vi "AutoIntakeRear.vi"() -> ()   [LabVIEW 2015]
uses:
  Typedef/IntakeControllerActions.ctl
  Typedef/IntakeControllerMsg.ctl
  ArmController/ArmController.lvlib
panel:
  in  "milliseconds to wait 2":u32=500
  in  "milliseconds to wait":u32=600
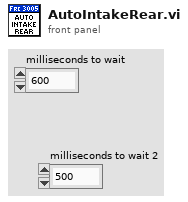
[diagram p1: front panel]
types:
  T1 = typedef "IntakeControllerMsg.ctl" = cluster{"Cmd":T2, "Data":variant}
  T2 = typedef "IntakeControllerActions.ctl" = enum16{"Wait on Intake Rear", "Wait on Angle Rear", "Go To Angle Rear", "Wait on Intake Front", "Wait on Angle Front", "Set Roller Front", "Set Roller Rear", "Go To Angle Front", "Wait ms"}
  T3 = cluster{"Down":dbl, "Pickup":dbl, "Shoot":dbl, "Turtle":dbl, "Intake Block":dbl, "Intake Transfer":dbl}
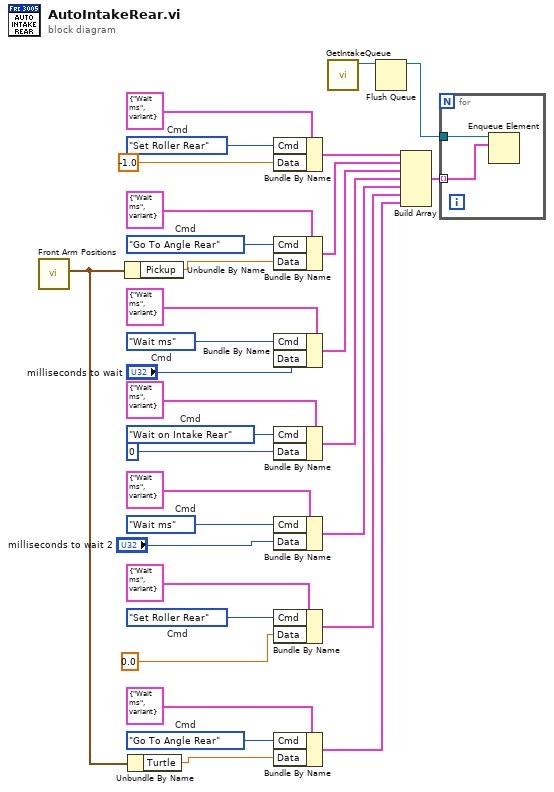
[diagram p0: block diagram]
diagram:
  w32 = IntakeControllerActions."Go To Angle Rear"  # Cmd
  w23 = IntakeControllerActions."Set Roller Rear"  # Cmd
  w27 = IntakeControllerActions."Wait ms"  # Cmd
  w20 = IntakeControllerActions."Wait on Intake Rear"  # Cmd
  w14 = IntakeControllerActions."Wait ms"  # Cmd
  w11 = IntakeControllerActions."Go To Angle Rear"  # Cmd
  w8 = IntakeControllerActions."Set Roller Rear"  # Cmd
  n1 = call "Front Arm Positions.vi"() -> ("Rear Arm"=w1:T3)  [unwired: 10 in, 1 out]
  n2 = Unbundle By Name(w1) -> ("Pickup"=w3:dbl)
  n3 = Unbundle By Name(w1) -> ("Turtle"=w2:dbl)
  n4 = Bundle By Name(cluster=T1 {"Cmd"=enum."Wait ms", "Data"=variant(i32 50)} ("output cluster"), "Cmd"=w8, "Data"=-1.0 ("Diffs")) -> (w10:T1)
  n5 = Bundle By Name(cluster=T1 {"Cmd"=enum."Wait ms", "Data"=variant(i32 50)} ("output cluster"), "Cmd"=w11, "Data"=w3) -> (w13:T1)
  n6 = Bundle By Name(cluster=T1 {"Cmd"=enum."Wait ms", "Data"=variant(i32 50)} ("output cluster"), "Cmd"=w14, "Data"="milliseconds to wait") -> (w17:T1)
  n7 = Bundle By Name(cluster=T1 {"Cmd"=enum."Wait ms", "Data"=variant(i32 50)} ("output cluster"), "Cmd"=w20, "Data"=u32 0 ("milliseconds to wait")) -> (w21:T1)
  n8 = Bundle By Name(cluster=T1 {"Cmd"=enum."Wait ms", "Data"=variant(i32 50)} ("output cluster"), "Cmd"=w27, "Data"="milliseconds to wait 2") -> (w29:T1)
  n9 = Bundle By Name(cluster=T1 {"Cmd"=enum."Wait ms", "Data"=variant(i32 50)} ("output cluster"), "Cmd"=w23, "Data"=0.0 ("Diffs")) -> (w30:T1)
  n10 = Bundle By Name(cluster=T1 {"Cmd"=enum."Wait ms", "Data"=variant(i32 50)} ("output cluster"), "Cmd"=w32, "Data"=w2) -> (w5:T1)
  n11 = call "GetIntakeQueue.vi"() -> ("queue out"=w6:refnum<queue>)  [unwired: 11 in]
  n12 = Flush Queue(queue=w6) -> (queue out=w4:refnum<queue>)  [unwired: 1 in, 2 out]
  n13 = Build Array(w10, w13, w17, w21, w29, w30, w5) -> (w22:T1[])
  n14 = for {
    tunnel: w4 -> [w34]
    tunnel: w22 -> [w33] mode=indexing
    n15 = Enqueue Element(queue=w34, element=w33) -> ()  [unwired: 2 in, 3 out]
  }
